vi "saveImages.vi"(7 "totalImageNumber":i32, 8 "error in (no error)":errorcluster, 9 "U16bit image data":u16[][](array[numeric]), 10 "Path":path, 11 "WinX32Camera in":refnum<class "WinX32Camera.lvclass">) -> (0 "error out":errorcluster, 3 "WinX32Camera out":refnum<class "WinX32Camera.lvclass">)   [LabVIEW 2011, in "WinX32Camera.lvclass"]
uses:
  WinX32Camera.lvclass
  WinX32Camera.lvclass/WinX32Camera.ctl
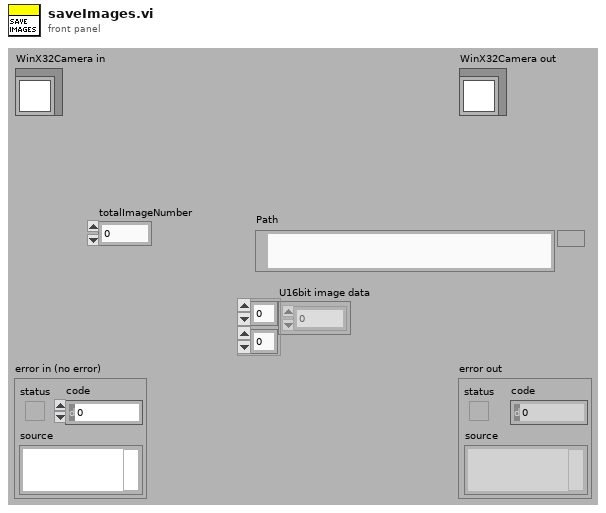
[diagram p1: front panel]
types:
  T1 = cluster{"cameraType":string, "imageName":string, "saved":string, "analysisType":string, "U16bit image data":u16[][], "path":path}
  T2 = typedef "Image Type" = u32
  T3 = typedef "IMAQ Image.ctl" = refnum<image>
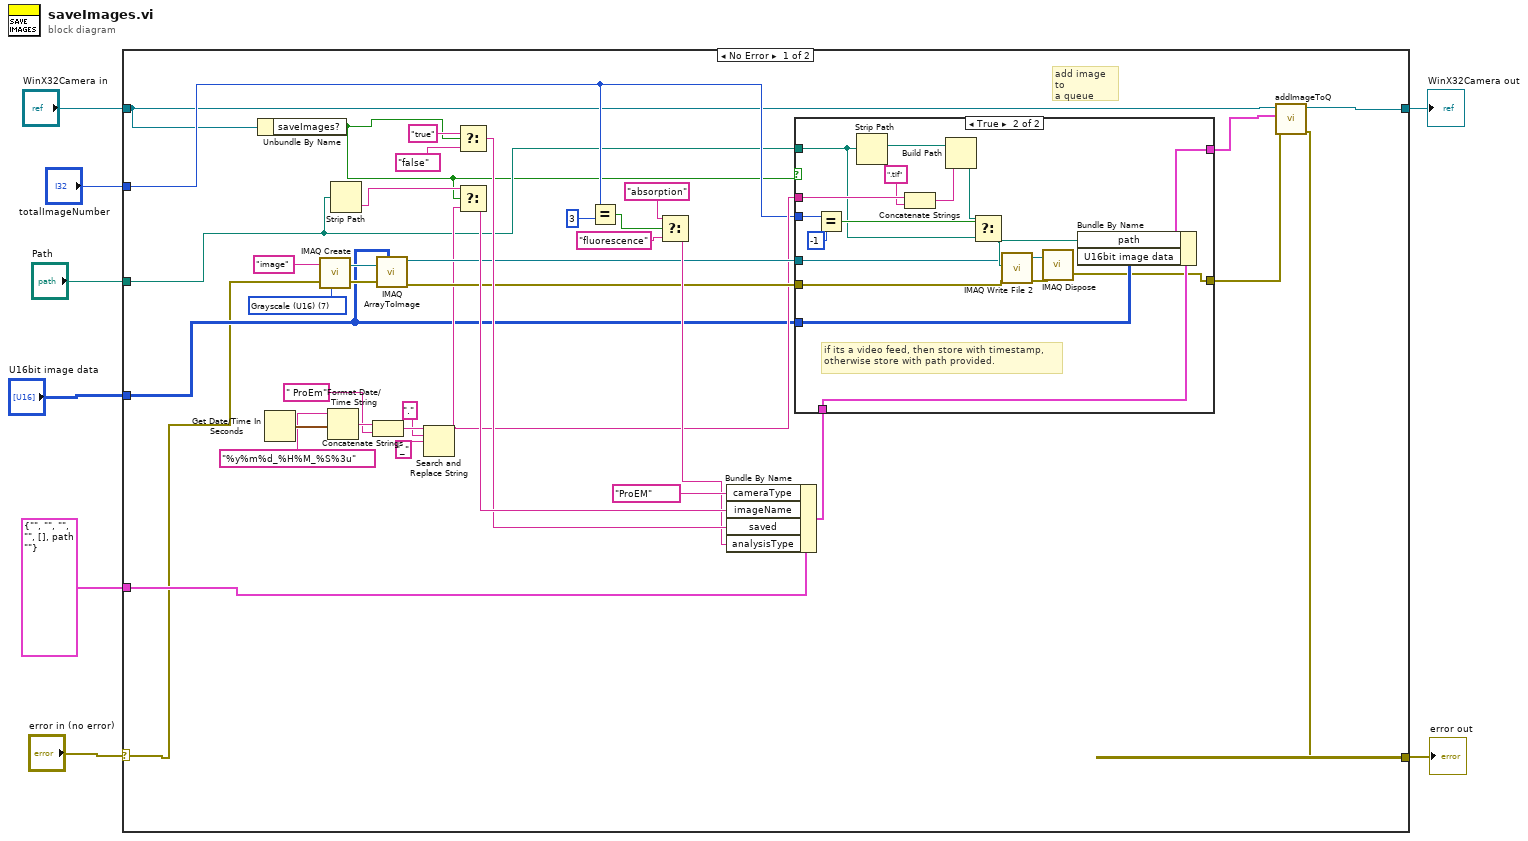
[diagram p0: block diagram]
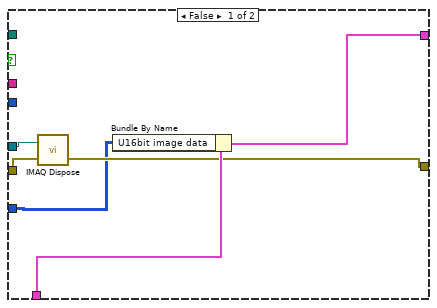
[diagram p2: hidden frame]
diagram:
  n1 = case shown="No Error" "error in (no error)" {
    selector: "error in (no error)" -> [w14 w71]
    tunnel: [w9 w71] -> w7
    tunnel: [w12 w70] -> w1
    tunnel: "WinX32Camera in" -> [w13 w70]
    tunnel: "totalImageNumber" -> [w19 _]
    tunnel: "U16bit image data" -> [w18 _]
    tunnel: "Path" -> [w17 _]
    tunnel: T1 {"cameraType"="", "imageName"="", "saved"="", "analysisType"="", "U16bit image data"=[], "path"=path ""} ("ImageData") -> [w16 _]
    frame No Error {
      w44 = T2 7 items=["Grayscale (U8)", "Grayscale (I16)", "Grayscale (SGL)", "Complex (CSG)", "RGB (U32)", "HSL (U32)", "RGB (U64)", "Grayscale (U16)"] ("Image Type")
      # "add image to\na queue"
      n2 = Unbundle By Name(w13) -> ("saveImages?"=w15:bool)
      n3 = Get Date/Time In Seconds() -> (seconds since 1Jan1904=w41:timestamp)
      n4 = call "IMAQ Create"("Image Name"="image", "Image Type"=w44, "error in (no error)"=w14) -> ("New Image"=w43:T3, "error out"=w42:errorcluster)  [unwired: 2 in]
      n5 = Format Date/Time String(time format string (%c)="%y%m%d_%H%M_%S%3u", seconds (now)=w41) -> (date/time string=w39:string)  [unwired: 1 in]
      n6 = Strip Path(path=w17) -> (name=w31:string)  [unwired: 1 out]
      n7 = Concatenate Strings(w39, " ProEm") -> (w23:string)
      n8 = call "IMAQ ArrayToImage"("Image Pixels (U16)"=w18, "error in (no error)"=w42, "Image"=w43) -> ("error out"=w24:errorcluster, "Image Out"=w25:T3)  [unwired: 7 in]
      n9 = Search and Replace String(input string=w23, search string=".", replace string="_") -> (result string=w22:string)  [unwired: 5 in, 3 out]
      n10 = Select(t="true", s=w15, f="false") -> (s? t:f=w28:string)
      n11 = Select(t=w31, s=w15, f=w22) -> (s? t:f=w29:string)
      n12 = Equal?(x=w19, y=3) -> (x = y?=w34:bool)
      n13 = Select(t="absorption", s=w34, f="fluorescence") -> (s? t:f=w27:string)
      n14 = Bundle By Name(cluster=w16, "cameraType"="ProEM", "imageName"=w29, "saved"=w28, "analysisType"=w27) -> (w26:T1)
      n15 = case shown="True" w15 {
        tunnel: [w49 w54] -> w10
        tunnel: [w50 w59] -> w11
        tunnel: w17 -> [_ w62]
        tunnel: w22 -> [_ w68]
        tunnel: w19 -> [_ w61]
        tunnel: w26 -> [w51 w60]
        tunnel: w18 -> [w48 w57]
        tunnel: w25 -> [w47 w53]
        tunnel: w24 -> [w46 w52]
        frame False {
          n16 = call "IMAQ Dispose"("Image"=w47, "error in (no error)"=w46) -> ("error out"=w49:errorcluster)  [unwired: 4 in]
          n17 = Bundle By Name(cluster=w51, "U16bit image data"=w48) -> (w50:T1)
        }
        frame True {
          # "if its a video feed, then store with timestamp,\notherwise store with path provided."
          n18 = Equal?(x=w61, y=-1) -> (x = y?=w63:bool)
          n19 = Strip Path(path=w62) -> (stripped path=w69:path)  [unwired: 1 out]
          n20 = Concatenate Strings(w68, ".tif") -> (w66:string)
          n21 = Build Path(base path=w69, name or relative path=w66) -> (appended path=w64:path)
          n22 = Select(t=w64, s=w63, f=w62) -> (s? t:f=w58:path)
          n23 = call-poly "IMAQ Write File 2"("error in (no error)"=w52, "File Path"=w58, "Image"=w53) -> ("error out"=w56:errorcluster, "Image Out (duplicate)"=w55:T3)  [unwired: 7 in]
          n24 = call "IMAQ Dispose"("Image"=w55, "error in (no error)"=w56) -> ("error out"=w54:errorcluster)  [unwired: 4 in]
          n25 = Bundle By Name(cluster=w60, "path"=w58, "U16bit image data"=w57) -> (w59:T1)
        }
      }
      n26 = call "addImageToQ.vi"("error in (no error)"=w10, "ImageData"=w11, "WinX32Camera in"=w13) -> ("error out"=w9:errorcluster, "WinX32Camera out"=w12:refnum<class "WinX32Camera.lvclass">)  [unwired: 7 in]
    }
    frame Error {
    }
  }
  "error out" <- w7
  "WinX32Camera out" <- w1
